vi "setPWM_NUM.vi"(8 "错误输入（无错误）":errorcluster, 10 "pulse num":dbl, 11 "axie":enum16{"x", "y"}(ring)) -> (0 "错误输出":errorcluster)   [LabVIEW 2013]
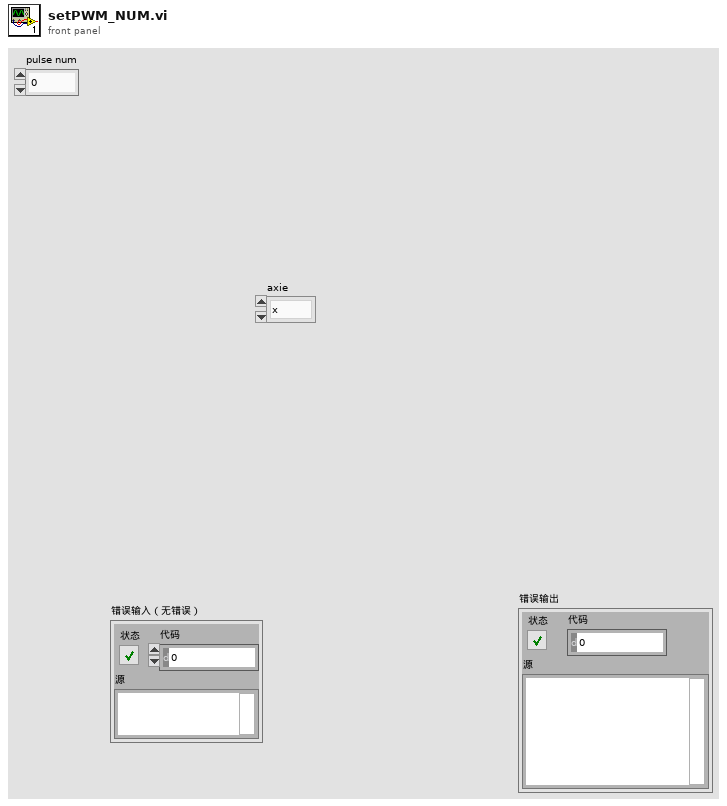
[diagram p1: front panel]
types:
  T1 = cluster{"cmd":string, "channel":i32, "value":dbl, "on/off":bool, "return value":refnum<vi>}
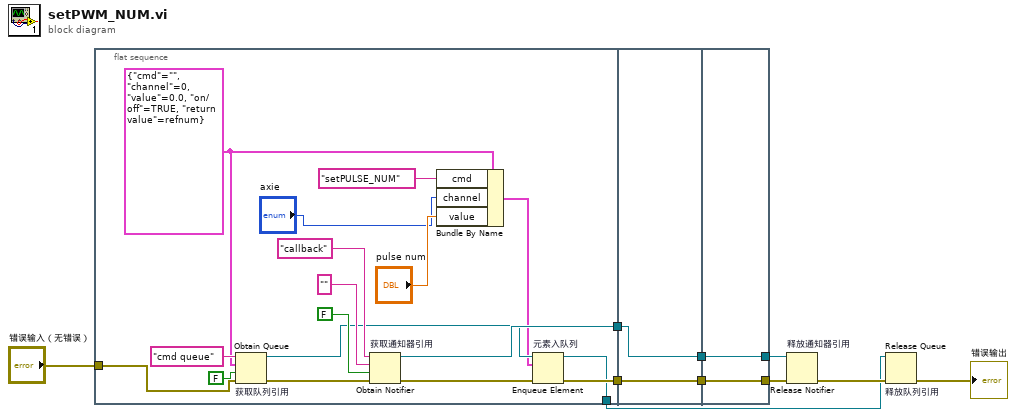
[diagram p0: block diagram]
diagram:
  n1 = flat-sequence {
    tunnel: [w24] -> w10
    tunnel: [w15] -> w5
    tunnel: [w14] -> w2
    tunnel: "错误输入（无错误）" -> [w13]
    tunnel: w10 -> [w28]
    tunnel: [w28] -> w9
    tunnel: [w29] -> w7
    tunnel: w5 -> [w29]
    tunnel: w9 -> [w31]
    tunnel: [w31] -> w8
    tunnel: w7 -> [w30]
    tunnel: [w30] -> w6
    frame #0 {
      w16 = T1 {"cmd"="", "channel"=0, "value"=0.0, "on/off"=TRUE, "return value"=refnum}
      n2 = Obtain Queue "获取队列引用"(name (unnamed)="cmd queue" ("名称（未命名）"), element data type=w16, create if not found? (T)=FALSE ("如未找到是否创建？(T)"), error in (no error)=w13) -> (queue out=w18:refnum<queue>, error out=w20:errorcluster)  [unwired: 1 in, 1 out]
      n3 = Obtain Notifier "获取通知器引用"(name (unnamed)="callback" ("名称（未命名）"), notification data type="", create if not found? (T)=FALSE ("如未找到是否创建？(T)"), error in (no error)=w20) -> (notifier out=w24:refnum<notifier>, error out=w19:errorcluster)  [unwired: 1 out]
      n4 = Bundle By Name(cluster=w16, "cmd"="setPULSE_NUM", "channel"="axie", "value"="pulse num") -> (w17:T1)
      n5 = Enqueue Element "元素入队列"(queue=w18, element=w17, error in (no error)=w19) -> (queue out=w14:refnum<queue>, error out=w15:errorcluster)  [unwired: 1 in, 1 out]
    }
    frame #1 {
    }
    frame #2 {
    }
  }
  n6 = Release Notifier "释放通知器引用"(notifier=w8, error in (no error)=w6) -> (error out=w4:errorcluster)  [unwired: 1 in, 2 out]
  n7 = Release Queue "释放队列引用"(queue=w2, error in (no error)=w4) -> (error out=→"错误输出":errorcluster)  [unwired: 1 in, 2 out]
